vi "NISE.Set NVMEM Bytes.vi"(0 "SLSC Interface in":refnum<class "SLSC Interface.lvclass">, 5 "NVMEM area":refnum<k21>="$DefaultNVMEMAreas", 7 "data address":u32 format="%.0x", 9 "data":u8[](array[numeric]) format="%.0x", 11 "error in (no error)":errorcluster) -> (4 "SLSC Interface out":refnum<class "SLSC Interface.lvclass">, 6 "NVMEM area out":refnum<k21>, 8 "next data address":u32 format="%.0x", 15 "error out":errorcluster)   [LabVIEW 2016, in "SLSC Interface.lvclass"]
uses:
  SLSC Interface.lvclass
panel:
  in  "session in":refnum<k21>
  out "session out":refnum<k21>
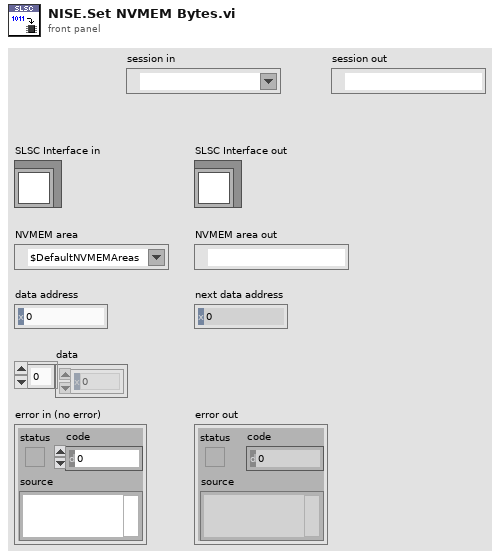
[diagram p1: front panel]
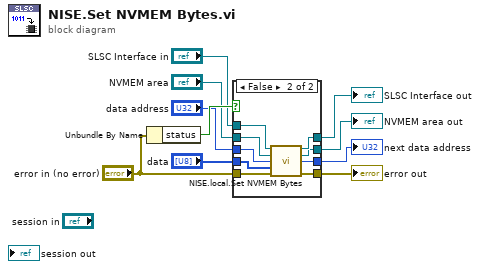
[diagram p0: block diagram]
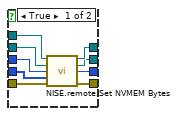
[diagram p2: hidden frame]
diagram:
  n1 = Unbundle By Name("error in (no error)") -> ("status"=w10:bool)
  n2 = case shown="False" w10 {
    tunnel: "SLSC Interface in" -> [w19 w28]
    tunnel: [w18 w27] -> w8
    tunnel: "NVMEM area" -> [w17 w26]
    tunnel: [w16 w25] -> w6
    tunnel: "data address" -> [w15 w24]
    tunnel: [w14 w23] -> w4
    tunnel: "data" -> [w13 w22]
    tunnel: "error in (no error)" -> [w12 w21]
    tunnel: [w11 w20] -> w1
    frame True {
      n3 = call "NISE.remote.Set NVMEM Bytes.vi"("SLSC Remote in"=w19, "NVMEM area"=w17, "data address"=w15, "data"=w13, "error in (no error)"=w12) -> ("SLSC Remote out"=w18:refnum<class "SLSC Interface.lvclass">, "NVMEM area out"=w16:refnum<k21>, "next data address"=w14:u32, "error out"=w11:errorcluster)  [unwired: 7 in]
    }
    frame False {
      n4 = call "NISE.local.Set NVMEM Bytes.vi"("SLSC Local in"=w28, "NVMEM area"=w26, "data address"=w24, "data"=w22, "error in (no error)"=w21) -> ("SLSC Local out"=w27:refnum<class "SLSC Interface.lvclass">, "NVMEM area out"=w25:refnum<k21>, "next data address"=w23:u32, "error out"=w20:errorcluster)  [unwired: 7 in]
    }
  }
  "error out" <- w1
  "SLSC Interface out" <- w8
  "next data address" <- w4
  "NVMEM area out" <- w6
